vi "Send.vi"(7 "Message Priority":T1, 8 "error in (no error)":errorcluster, 10 "Message":refnum<class "Message Interface.lvclass">, 11 "Message Transport Queue":refnum<class "Message Transport Queue.lvclass">) -> (0 "error out":errorcluster)   [LabVIEW 2016, in "WebSocket Networking.lvlib" / "WSserver Command Response Msg.lvclass"]
doc: "--\nCopyright © 2017 Composed SystemsI All rights reserved.\n\nAuthor: Jon McBee <jon.mcbee@composed.io>\n\nThis library is provided \"AS IS\" ,WITHOUT WARRANTIES OR\nCONDITIONS OF ANY KIND, either express or implied.\n\nComposed Systems -- composed.io\n\nStream 0.0.1.1\nJon McBee - Composed Systems\nCopyright (c) 2017, Composed Systems"
uses:
  <userlib>/Common Components/WebSocket Networking/WS Server Msgs/WSserver Command Response Msg/WSserver Command Response Msg.lvclass
  <userlib>/Composed Systems/Stream/Mediator/Classes/Message Transport Queue/Message Transport Queue.lvclass
  <userlib>/Composed Systems/Stream/Mediator/Classes/Message Transport Interface/Message Priority.ctl
  <userlib>/Composed Systems/Stream/Mediator/Classes/Message Interface/Message Interface.lvclass
  C:/Program Files (x86)/National Instruments/LabVIEW 2016/user.lib/Composed Systems/Stream/Mediator/Classes/Message Interface/Message Interface.lvclass
  <userlib>/Common Components/WebSocket Networking/WS Server Msgs/WSserver Command Response Msg/WSserver Command Response Msg.lvclass/WSserver Command Response Msg.ctl
  <userlib>/Composed Systems/Stream/Mediator/Classes/Message Transport Interface/Message Transport Interface.lvclass
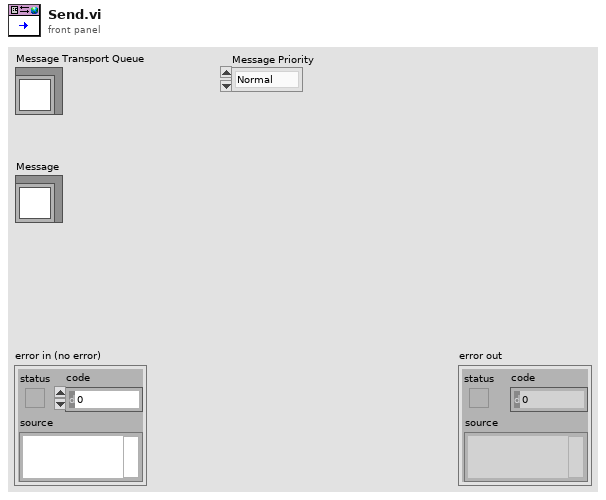
[diagram p1: front panel]
types:
  T1 = typedef "Stream Mediator.lvlib/Message Transport Interface.lvclass/Message Priority.ctl" = enum16{"Normal", "High"}
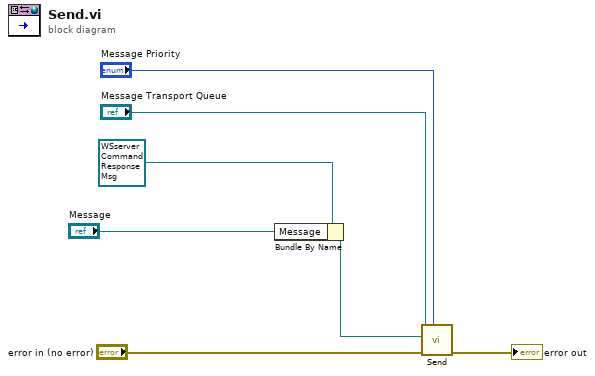
[diagram p0: block diagram]
diagram:
  n1 = Bundle By Name(cluster=refnum<class "WSserver Command Response Msg.lvclass"> refnum ("WSserver Command Dispatch Msg.lvclass"), "Message"="Message") -> (w4:refnum<class "WSserver Command Response Msg.lvclass">)
  n2 = call-dynamic "Send.vi"("Message Priority"="Message Priority", "error in (no error)"="error in (no error)", "Message"=w4, "Message Transport Queue in"="Message Transport Queue") -> ("error out"=→"error out":errorcluster)  [unwired: 5 in, 2 out]
